vi "reformulaçaoAtacante.vi"(9 "balls":T7[](array[typedef]), 10 "Robot in":T1, 11 "IA State":T6={"our_robots"=[], "enemy_robots"=[], "balls"=[], "geometry"={"field_length"=0, "field_width"=0, "goal_width"=0, "goal_depth"=0, "center_circle_radius"=0, "defense_width"=0, "defense_depth"=0, "free_kick_from_defense_dist"=0, "penalty_spot_from_field_line_dist"=0, "penalty_line_from_spot_dist"=0, "half_moon_depth"=0, "half_moon_width"=0}, "IA Judge"={"stage"="", "command"="", "our_goalie_id"=0.0, "enemy_goalie_id"=0.0, "command enum"=enum."Halt", "Time"=enum."Azul"}, "Received Timestamp"=timestamp(0 s since 1904-01-01), "Events"={"Touch"=FALSE, "id touch"=0.0, "Ball out of \nVision"=FALSE, "Ball inside \nGoalie area"=FALSE, "Robot not responding"=FALSE, "Robots responding status"=[1.0, 1.0, 1.0, 1.0, 1.0, 1.0], "Enemy Ball \nPossession"=FALSE, "Id ini Possession"=0.0, "Ball Possesion"=FALSE, "Id Possesion"=0.0, "Ball at\nour goal side"=FALSE, "Ball at\ntouchline"=FALSE, "Ball at\nenemy goal side"=FALSE}}) -> (3 "Robot out":T1)   [LabVIEW 2018]
uses:
  Intel/Functions Enum.ctl
  Intel/AttackerStates.ctl
  Path Planning/RRT/PathDest.ctl
  Path Planning/RRT/PathDests.ctl
  Core/AI Robot.ctl
  Core/AI Ball.ctl
  Core/Field Size.ctl
  Intel/Command Enum.ctl
  Core/AI Judge.ctl
  Util/Events/Events.ctl
  Core/AI Input.ctl
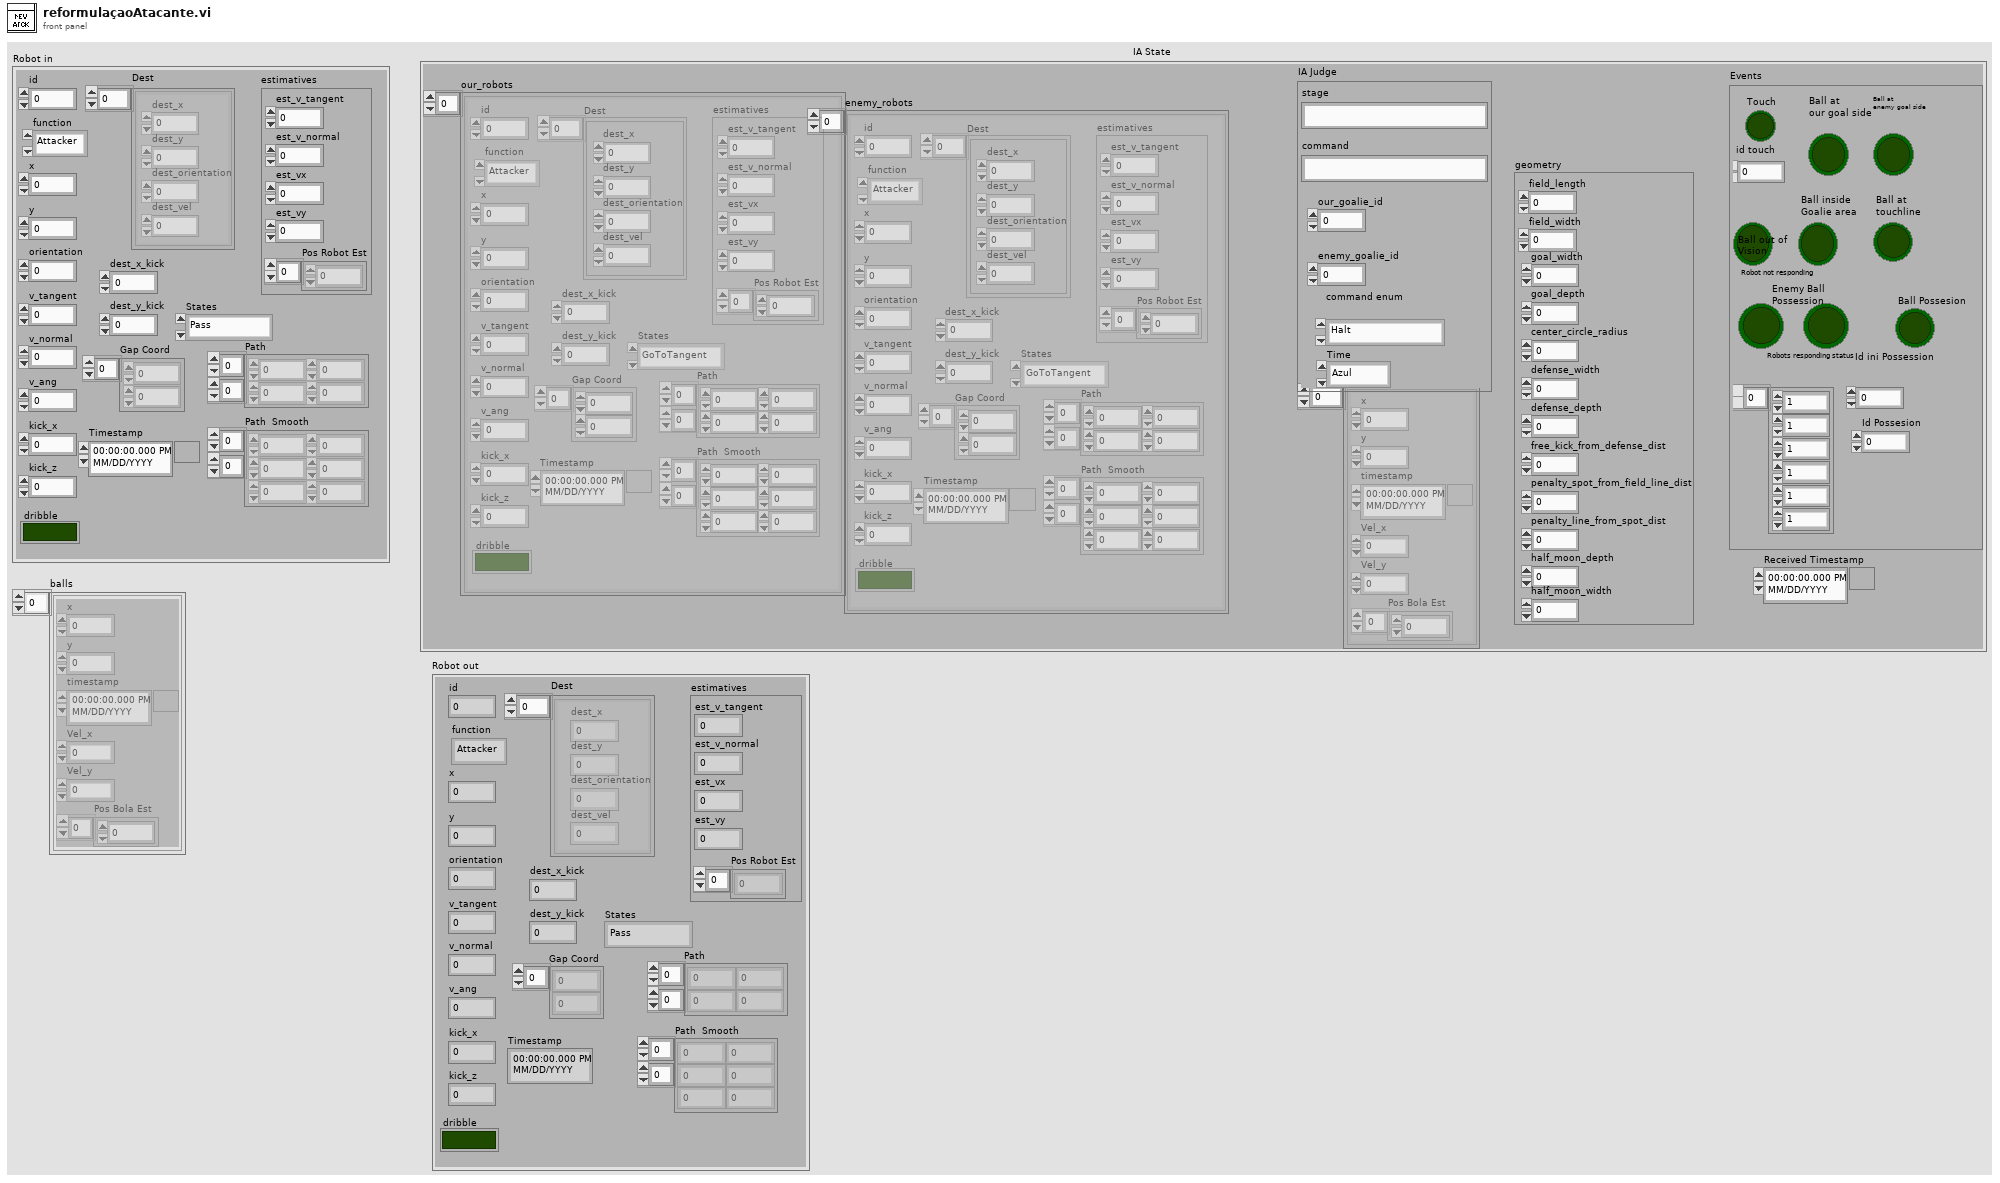
[diagram p1: front panel]
types:
  T1 = typedef "AI Robot.ctl" = cluster{"id":u32, "function":T2, "x":dbl, "y":dbl, "orientation":dbl, "v_tangent":dbl, "v_normal":dbl, "v_ang":dbl, "kick_x":dbl, "kick_z":dbl, "dribble":bool, "Timestamp":timestamp, "estimatives":cluster{"est_v_tangent":dbl, "est_v_normal":dbl, "est_vx":dbl, "est_vy":dbl, "Pos Robot Est":dbl[]}, "dest_x_kick":dbl, "dest_y_kick":dbl, "Gap Coord":dbl[], "States":T3, "Path ":dbl[][], "Path  Smooth":dbl[][], "Dest":T4}
  T2 = typedef "Functions Enum.ctl" = enum16{"Attacker", "Goalie", "Defender", "Striker", "Goto 0", "Dummy", "Kicker", "ZigZag"}
  T3 = typedef "AttackerStates.ctl" = enum16{"Pass", "GoToTangent", "BallGetting", "GoToKick", "Rotate anti-clockwise", "Rotate Clockwise", ""}
  T4 = typedef "PathDests.ctl" = T5[]
  T5 = typedef "PathDest.ctl" = cluster{"dest_x":dbl, "dest_y":dbl, "dest_orientation":dbl, "dest_vel":dbl}
  T6 = typedef "AI Input.ctl" = cluster{"our_robots":T1[], "enemy_robots":T1[], "balls":T7[], "geometry":T8, "IA Judge":T9, "Received Timestamp":timestamp, "Events":T11}
  T7 = typedef "AI Ball.ctl" = cluster{"x":dbl, "y":dbl, "timestamp":timestamp, "Vel_x":dbl, "Vel_y":dbl, "Pos Bola Est":dbl[]}
  T8 = typedef "Field Size.ctl" = cluster{"field_length":u32, "field_width":u32, "goal_width":u32, "goal_depth":u32, "center_circle_radius":u32, "defense_width":u32, "defense_depth":u32, "free_kick_from_defense_dist":u32, "penalty_spot_from_field_line_dist":u32, "penalty_line_from_spot_dist":u32, "half_moon_depth":u32, "half_moon_width":u32}
  T9 = typedef "AI Judge.ctl" = cluster{"stage":string, "command":string, "our_goalie_id":dbl, "enemy_goalie_id":dbl, "command enum":T10, "Time":enum16{"Azul", "Amarelo"}}
  T10 = typedef "Command Enum.ctl" = enum16{"Halt", "Stop", "Force Start", "PKA Normal Start", "Prepare Kickoff Ally", "PKE Normal Start", "Prepare Kickoff Enemy", "Prepare Penalty Ally", "PPA Normal Start", "Prepare Penalty Enemy", "PPE Normal Start", "Ball Placement Enemy Up", "Ball Placement Enemy Down", "Ball Placement Ally Up", "Ball Placement Ally Mid", "Ball Placement Ally Down", "Indirect Free Enemy", "Indirect Free Ally", "Timeout Enemy", "Timeout Ally", "Goal Enemy", "Goal Ally", "Normal Half Time", "Extra Time Break", "Extra Half Time", "None", "Post Game"}
  T11 = typedef "Events.ctl" = cluster{"Touch":bool, "id touch":dbl, "Ball out of \nVision":bool, "Ball inside \nGoalie area":bool, "Robot not responding":bool, "Robots responding status":dbl[], "Enemy Ball \nPossession":bool, "Id ini Possession":dbl, "Ball Possesion":bool, "Id Possesion":dbl, "Ball at\nour goal side":bool, "Ball at\ntouchline":bool, "Ball at\nenemy goal side":bool}
  T12 = enum16{"None", "Frente", "Trás", "Cima", "Baixo"}
  T13 = enum16{"Fazer gol pela lateral", "Tirar bola da parede", "Default", "Sair da parede", "Spin igual a um louco"}
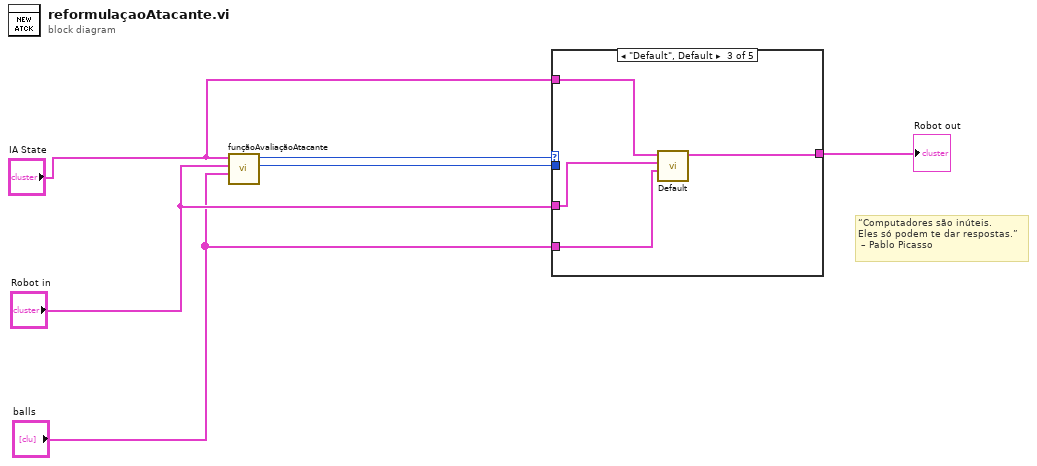
[diagram p0: block diagram]
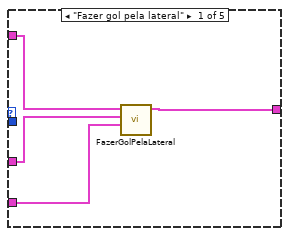
[diagram p2: hidden frame]
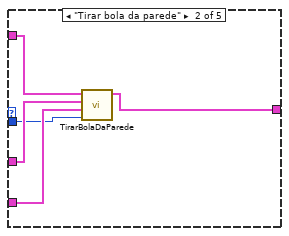
[diagram p3: hidden frame]
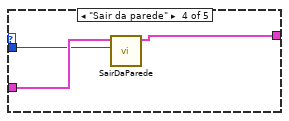
[diagram p4: hidden frame]
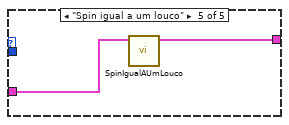
[diagram p5: hidden frame]
diagram:
  # "“Computadores são inúteis.\nEles só podem te dar respostas.”\n – Pablo Picasso"
  n1 = call "funçãoAvaliaçãoAtacante.vi"("balls"="balls", "Robot in"="Robot in", "IA State"="IA State") -> ("Parede"=w4:T12, "Estado_Atacante"=w6:T13)  [unwired: 7 in]
  n2 = case shown="\"Default\", Default" w6 {
    tunnel: "Robot in" -> [w9 w14 w18 w22 w24]
    tunnel: [w7 w11 w16 w20 w23] -> w1
    tunnel: w4 -> [_ w12 _ w21 _]
    tunnel: "IA State" -> [w10 w15 w19 _ _]
    tunnel: "balls" -> [w8 w13 w17 _ _]
    frame "Fazer gol pela lateral" {
      n3 = call "FazerGolPelaLateral.vi"("balls"=w8, "Robot in"=w9, "IA State"=w10) -> ("Cluster de saída"=w7:T1)  [unwired: 8 in]
    }
    frame "Tirar bola da parede" {
      n4 = call "TirarBolaDaParede.vi"("Parede"=w12, "balls"=w13, "Robot in"=w14, "IA State"=w15) -> ("Cluster de saída"=w11:T1)  [unwired: 7 in]
    }
    frame "Default", Default {
      n5 = call "Default.vi"("balls"=w17, "Robot in"=w18, "IA State"=w19) -> ("Cluster de saída"=w16:T1)  [unwired: 8 in]
    }
    frame "Sair da parede" {
      n6 = call "SairDaParede.vi"("Parede"=w21, "Robot in"=w22) -> ("Cluster de saída"=w20:T1)  [unwired: 9 in]
    }
    frame "Spin igual a um louco" {
      n7 = call "SpinIgualAUmLouco.vi"("Robot in"=w24) -> ("Cluster de saída"=w23:T1)  [unwired: 10 in]
    }
  }
  "Robot out" <- w1
